vi "emi_Defer Panel Updates OFF(w.cursor).vi"(5 "VI Refnum(This VI)":refnum<vi>, 9 "error in (no error)":errorcluster) -> (6 "VI Refnum Out":refnum<vi>, 10 "error out":errorcluster)   [LabVIEW 2011]
doc: "Gets a vi panel refrence, sets defere panel update to true, close panel refrence.\n\nIf not VI Refnum in, the refrence of the vi where this funciton is used is employed, and subsequently closed. (If refrence not explisitly vired, it does not need to be closed)\n\nIf error in: Perform action anyway\nIf error Still tries to turn off defere panel up date, if this generates error, it is put in Error out if no other error."
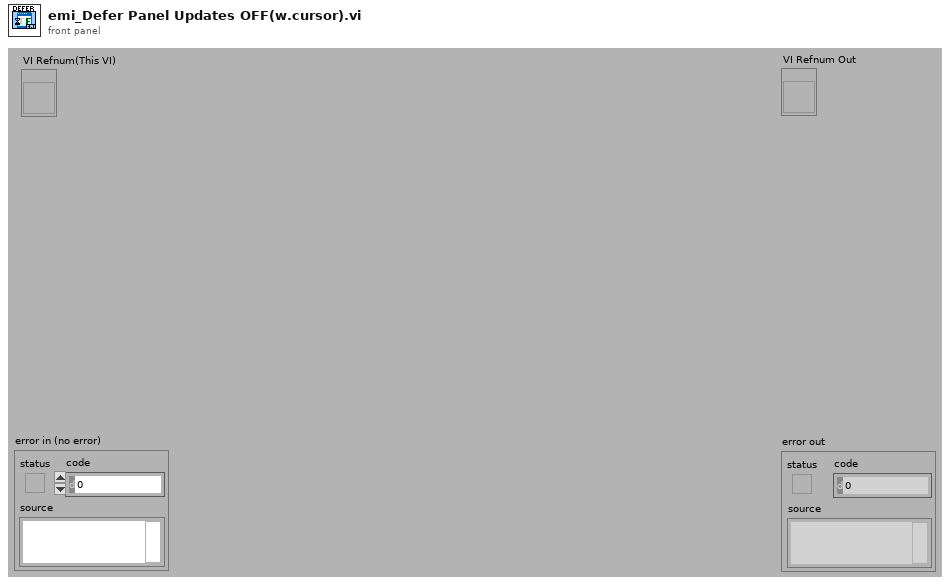
[diagram p1: front panel]
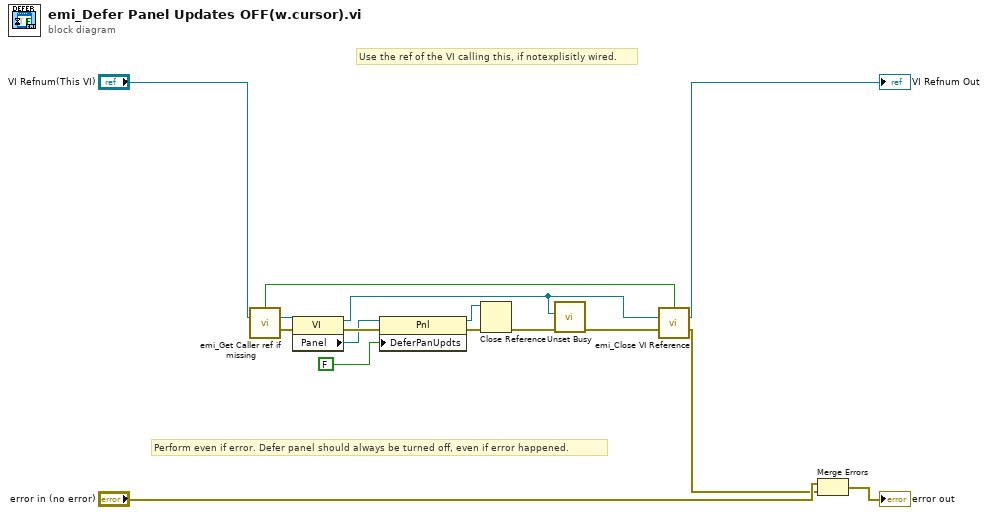
[diagram p0: block diagram]
diagram:
  # "Perform even if error. Defer panel should always be turned off, even if error happened."
  # "Use the ref of the VI calling this, if notexplisitly wired."
  n1 = call "emi_Get Caller ref if missing.vi"("VI Refnum(Calling VI)"="VI Refnum(This VI)") -> ("Ref Generated"=w11:bool, "VI Refnum Out"=w3:refnum<vi>, "error out"=w6:errorcluster)  [unwired: 12 in]
  n2 = property class="VI"(reference=w3, error in=w6) -> (reference out=w1:refnum<vi>, error out=w15:errorcluster, "Panel"=w14:refnum<vi>)
  n3 = property class="Pnl"(reference=w14, error in=w15, "DeferPanUpdts"=FALSE ("Defer Panel Updates")) -> (reference out=w13:refnum<vi>, error out=w12:errorcluster)
  n4 = Close Reference(reference=w13, error in (no error)=w12) -> (error out=w7:errorcluster)
  n5 = call <vilib>:"Unset Busy.vi"("error in (no error)"=w7, "VI reference (current VI)"=w1) -> ("error out"=w2:errorcluster)  [unwired: 9 in]
  n6 = call "emi_Close VI Reference.vi"("Close ref?(T)"=w11, "VI Refnum"=w1, "error in (no error)"=w2) -> ("VI Refnum Out"=→"VI Refnum Out":refnum<vi>, "error out"=w8:errorcluster)  [unwired: 11 in]
  n7 = Merge Errors("error in (no error)", w8) -> (→"error out":errorcluster)
